vi "wczytać_plik.vi"(8 "error in":errorcluster, 11 "wejœcie cluster":T1={"Runer's Data"={"Name"="", "Age"=0}, "HR Max"=0, "Raw Data"={"Time"=[], "Bpm"=[]}, "% HR MAX "=[], "HR Zones "=[], "no of points"=[], "Heart Rate Zone No 2"=[1, 2, 3, 4, 5]}) -> (0 "error  out":errorcluster, 3 "wyjœcie cluster":T1={"Runer's Data"={"Name"="", "Age"=0}, "HR Max"=0, "Raw Data"={"Time"=[], "Bpm"=[]}, "% HR MAX "=[], "HR Zones "=[], "no of points"=[], "Heart Rate Zone No 2"=[1, 2, 3, 4, 5]})   [LabVIEW 2024]
uses:
  klaster 2.ctl
  klaster.ctl
  klaster 4.ctl
  <vilib>/JDP Science/JDP Science Common Utilities/Timestamp/JDP Timestamp.lvlib
panel:
  out "text":string
  in  "file path (use dialog)":path
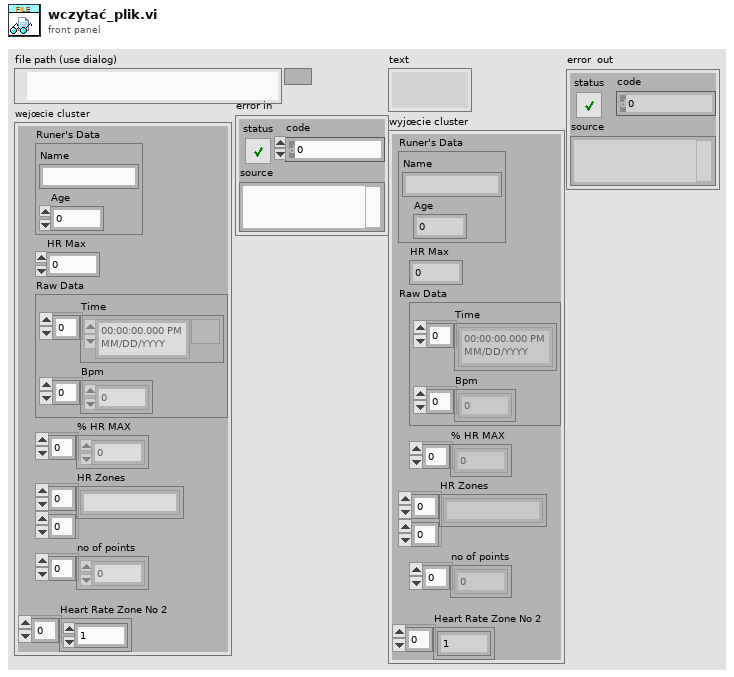
[diagram p1: front panel]
types:
  T1 = typedef "klaster 4.ctl" = cluster{"Runer's Data":T2, "HR Max":i32, "Raw Data":T3, "% HR MAX ":dbl[], "HR Zones ":string[][], "no of points":dbl[], "Heart Rate Zone No 2":i32[]}
  T2 = typedef "klaster.ctl" = cluster{"Name":string, "Age":i32}
  T3 = typedef "klaster 2.ctl" = cluster{"Time":timestamp[], "Bpm":i32[]}
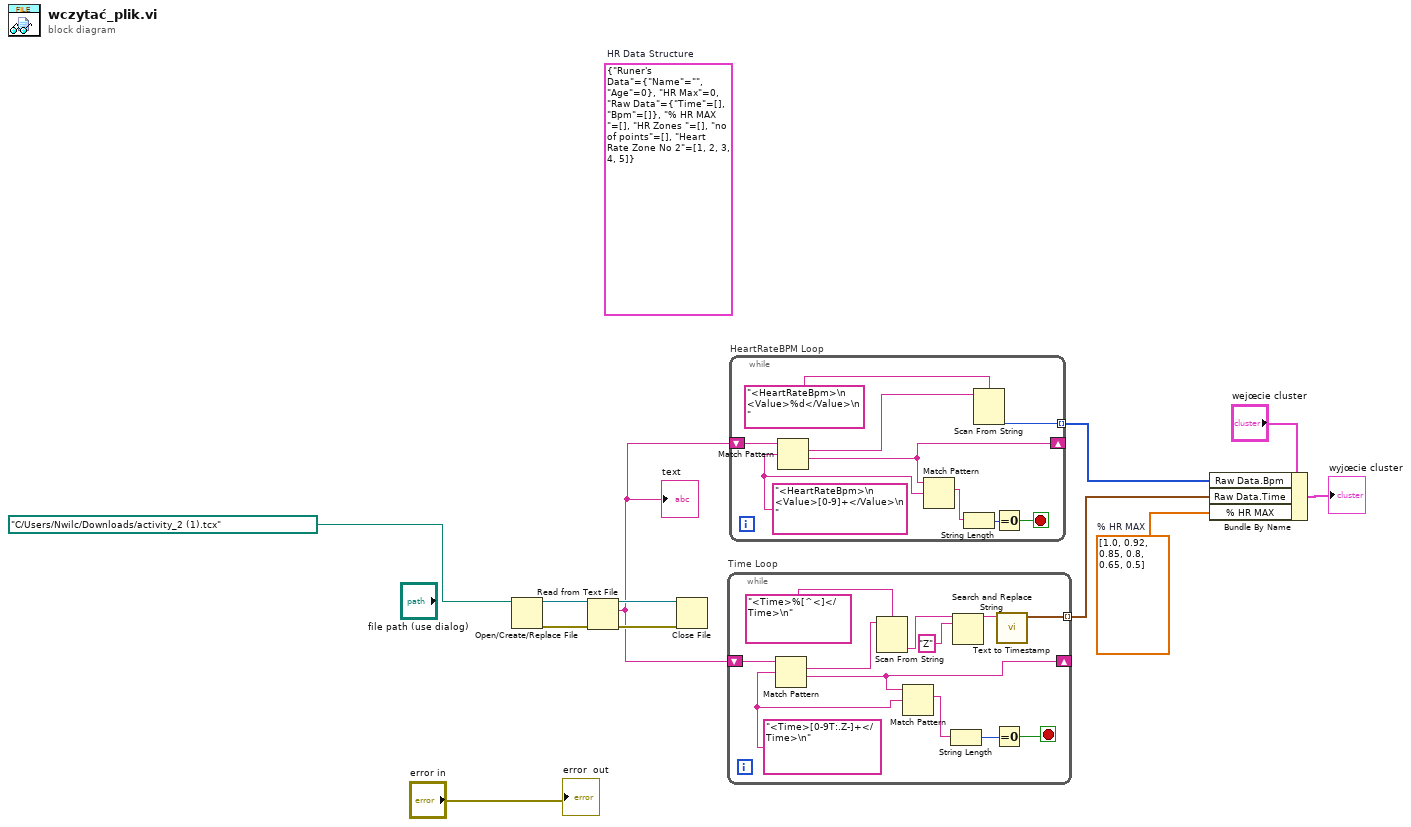
[diagram p0: block diagram]
diagram:
  w1 = dbl[] [1.0, 0.92, 0.85, 0.8, 0.65, 0.5]  # % HR MAX
  (unwired) T1 {"Runer's Data"={"Name"="", "Age"=0}, "HR Max"=0, "Raw Data"={"Time"=[], "Bpm"=[]}, "% HR MAX "=[], "HR Zones "=[], "no of points"=[], "Heart Rate Zone No 2"=[1, 2, 3, 4, 5]}  # HR Data Structure
  n1 = Open/Create/Replace File(file path (use dialog)=path "C:/Users/Nwilc/Downloads/activity_2 (1).tcx") -> (refnum out=w12:refnum<file>, error out=w11:errorcluster)  [unwired: 5 in, 1 out]
  n2 = Read from Text File(file (use dialog)=w12, error in=w11) -> (refnum out=w9:refnum<file>, text=w2:string, error out=w10:errorcluster)  [unwired: 2 in, 1 out]
  "text" <- w2
  n3 = Close File(refnum=w9, error in=w10) -> ()  [unwired: 2 out]
  n4 = while "Time Loop" {
    shift-right: [w17] -> _
    shift-left: w2 -> [w23]
    tunnel: [w18] -> w6 mode=indexing
    stop <- w13 stop-if-true
    w16 = "<Time>[0-9T:.Z-]+</Time>\n" ("regular expression")
    n5 = Match Pattern(string=w23, regular expression=w16) -> (match substring=w21:string, after substring=w17:string)  [unwired: 1 in, 2 out]
    n6 = Scan From String(format string="<Time>%[^<]</Time>\n", input string=w21) -> (output 1=w20:string)  [unwired: 3 in, 3 out]
    n7 = Match Pattern(string=w17, regular expression=w16) -> (match substring=w15:string)  [unwired: 1 in, 3 out]
    n8 = String Length(string=w15) -> (length=w14:i32)
    n9 = Search and Replace String(input string=w20, search string="Z" ("replace string (\"\")")) -> (result string=w19:string)  [unwired: 6 in, 3 out]
    n10 = Equal To 0?(x=w14) -> (x = 0?=w13:bool)
    n11 = call <vilib>:"Text to Timestamp.vi"("Text Timestamp"=w19) -> ("Time Stamp"=w18:timestamp)  [unwired: 7 in, 3 out]
  }
  n12 = while "HeartRateBPM Loop" {
    tunnel: [w30] -> w3 mode=indexing
    shift-right: [w29] -> _
    shift-left: w2 -> [w32]
    stop <- w25 stop-if-true
    w28 = "<HeartRateBpm>\n              <Value>[0-9]+</Value>\n          " ("regular expression")
    n13 = Match Pattern ("Match Pattern -BPM")(string=w32, regular expression=w28) -> (match substring=w31:string, after substring=w29:string)  [unwired: 1 in, 2 out]
    n14 = Match Pattern ("Match Pattern -BPM")(string=w29, regular expression=w28) -> (match substring=w27:string)  [unwired: 1 in, 3 out]
    n15 = String Length(string=w27) -> (length=w26:i32)
    n16 = Scan From String(format string="<HeartRateBpm>\n              <Value>%d</Value>\n            ", input string=w31) -> (output 1=w30:i32)  [unwired: 3 in, 3 out]
    n17 = Equal To 0?(x=w26) -> (x = 0?=w25:bool)
  }
  n18 = Bundle By Name(cluster="wejœcie cluster", "Raw Data.Bpm"=w3, "Raw Data.Time"=w6, "% HR MAX"=w1) -> (→"wyjœcie cluster":T1)
  "error  out" <- "error in"
